vi "Autonomous.vi"   [LabVIEW 2023]
doc: "This VI starts when autonomous period begins, and will automatically be terminated when it ends. You can carry out timed or sensor driven operations directly to I/O or to subsystems without needing to return to the caller."
uses:
  <vilib>/Rock Robotics/WPI/ThirdParty/JAS_Junk/TrajLib/Trajectory_Library.lvlib
  <vilib>/Rock Robotics/WPI/ThirdParty/MJansen/PathPlanner/PathPlanner24.lvlib
  <vilib>/Rock Robotics/WPI/ThirdParty/JAS_Junk/TrajLib/TypeDef/CHASSIS_SPEEDS.ctl
  <vilib>/Rock Robotics/Network Tables/NT Read String.vi
types:
  T1 = typedef "Trajectory_Library.lvlib/CHASSIS_SPEEDS.ctl" = cluster{"vX":dbl, "vY":dbl, "vOmega":dbl}
  T2 = typedef "WPI_JoystickDevRef.ctl" = cluster{"Device":T3}
  T3 = typedef "WPI_JoystickDeviceEnum.ctl" = enum16{"USB 0", "USB 1", "USB 2", "USB 3", "USB 4", "USB 5"}
  T4 = typedef "WPI_MotorControlDeviceRef.ctl" = cluster{"DeviceStatus":errorcluster, "Type":T5, "PWM":cluster{"PWM Channel":T6, "DeadBand":T7}, "CAN":cluster{"Device Number":u8, "SetOutput VI Ref":variant, "GetOutput VI Ref":variant, "Enable VI Ref":variant, "Disable VI Ref":variant, "Data":variant}, "Invert":bool, "DIO PWM":cluster{"PWM \"Enable\" Channel":T6, "DIOChannel":T8, "PWM Rate":dbl}}
  T5 = typedef "WPI_MotorControlType.ctl" = enum16{"PWM", "CAN", "DIO PWM"}
  T6 = typedef "FPGA_DIOPWMChannel.ctl" = enum8{"PWM 0", "PWM 1", "PWM 2", "PWM 3", "PWM 4", "PWM 5", "PWM 6", "PWM 7", "PWM 8", "PWM 9", "PWM MXP 0", "PWM MXP 1", "PWM MXP 2", "PWM MXP 3", "PWM MXP 4", "PWM MXP 5", "PWM MXP 6", "PWM MXP 7", "PWM MXP 8", "PWM MXP 9", "Invalid"}
  T7 = typedef "WPI_PWMDeadband.ctl" = cluster{"Name":string, "maxPositivePwm":i32, "minPositivePwm":i32, "centerPwm":i32, "maxNegativePwm":i32, "minNegativePwm":i32, "angularRange":u16}
  T8 = typedef "FPGA_DIOChannel.ctl" = enum8{"DIO 0", "DIO 1", "DIO 2", "DIO 3", "DIO 4", "DIO 5", "DIO 6", "DIO 7", "DIO 8", "DIO 9", "DIO MXP 0", "DIO MXP 1", "DIO MXP 2", "DIO MXP 3", "DIO MXP 4", "DIO MXP 5", "DIO MXP 6", "DIO MXP 7", "DIO MXP 8", "DIO MXP 9", "DIO MXP 10", "DIO MXP 11", "DIO MXP 12", "DIO MXP 13", "DIO MXP 14", "DIO MXP 15", "SPI Port CS1", "SPI Port CS2", "SPI Port CS3", "SPI Port MISO", "SPI Port MOSI", "Invalid"}
  T9 = typedef "Trajectory_Library.lvlib/ROTATION2D.ctl" = cluster{"VALUE":dbl, "COS":dbl, "SIN":dbl}
  T10 = typedef "Trajectory_Library.lvlib/SWERVE_DRIVE_MODULE_POSITION.ctl" = cluster{"Distance":dbl, "Angle":T9, "P":bool}
  T11 = typedef "PathPlanner24.lvlib/PathPlannerPath.ctl" = cluster{"BezierPoints":T12[], "PreviewStartingRotation":T9, "Reversed":bool, "RotationTargets":T13[], "ConstraintZones":T14[], "EventMarkers":T16[], "GlobalConstraints":T15, "GoalEndState":T19, "AllPoints":T20[]}
  T12 = typedef "Trajectory_Library.lvlib/TRANSLATION2D.ctl" = cluster{"X":dbl, "Y":dbl}
  T13 = typedef "PathPlanner24.lvlib/PathPlannerRotationTarget.ctl" = cluster{"target":T9, "WaypointRelativePosition":dbl, "Exists":bool}
  T14 = typedef "PathPlanner24.lvlib/PathPlannerConstraintsZone.ctl" = cluster{"minWaypointPos":dbl, "maxWaypointPos":dbl, "Constraints":T15, "Present":bool}
  T15 = typedef "PathPlanner24.lvlib/PathPlannerPathConstraints.ctl" = cluster{"MaxVelocityMps;":dbl, "MaxAccelerationMpsSq;":dbl, "MaxAngularVelRadPsEc;":dbl, "MaxAngularAccRadPSecSq":dbl, "Exists":bool}
  T16 = typedef "PathPlanner24.lvlib/PathPlannerEventMarker.ctl" = cluster{"WaypointRelativePos":dbl, "minimumTriggerDistance":dbl, "markerPos":T12, "lastRobotPos":T12, "Command":T17, "markerPos Exists":bool, "LastRobotPoseExists":bool, "Triggered":bool}
  T17 = typedef "PathPlanner24.lvlib/PathPlannerCommandUtil.ctl" = cluster{"waitTime":dbl, "name":string, "pathName":string, "commands":cluster{"type":T18, "waitTime":dbl, "name":string, "pathName":string}[], "type":T18}
  T18 = typedef "PathPlanner24.lvlib/PathPlanner_CommandUtilType_ENUM.ctl" = enum16{"Unknown", "Wait", "Named", "Path", "Sequential", "Parallel", "Race", "Deadline"}
  T19 = typedef "PathPlanner24.lvlib/PathPlannerGoalEndState.ctl" = cluster{"Velocity":dbl, "Rotation":T9}
  T20 = typedef "PathPlanner24.lvlib/PathPlannerPathPoint.ctl" = cluster{"Position":T12, "HolonomicRotation":T9, "DistAlongPath":dbl, "CurveRadius":dbl, "MaxV":dbl, "Constraints":T15, "HolonomicRotationExists":bool}
  T21 = typedef "ADIS16470 Device Reference.ctl" = cluster{"DevStatus":errorcluster, "Hardware Config":T22, "Calibration Complete":refnum<notifier>, "Status Reference":refnum<data-value>, "Data Reference":refnum<data-value>, "Sychronous Process VI":T25, "Cmd FIFO":refnum<k33>, "Source":T26, "Data FIFO":refnum<k33>, "Calibration Time (ms)":u32, "Data Reference":refnum<data-value>}
  T22 = typedef "ADIS16470 Hardware Configuration.ctl" = cluster{"SPI Clock Rate (Hz)":dbl, "IMU SPI Mode (3)":T23, "IMU Reset Pin":T8, "IMU SPI Bus":T24, "IMU Data Ready Pin":T8, "Stall Config":cluster{"Pow2BytesPerRead":u8, "StallTicks":u16, "CsToSclkTicks":u8}}
  T23 = typedef "WPI_SPIMode.ctl" = enum16{"Mode 0 (Clk Idle Low,Sample on Leading)", "Mode 1 (Clk Idle Low,Sample on Trailing)", "Mode 2 (Clk Idle High,Sample on Leading)", "Mode 3 (Clk Idle High,Sample on Trailing)"}
  T24 = typedef "spi_bus.ctl" = enum16{"SPI On-Board, CS0", "SPI On-Board, CS1", "SPI On-Board, CS2", "SPI On-Board, CS3", "SPI MXP", "Invalid"}
  T25 = typedef "ADIS16470 Process.ctl" = refnum<vi>
  T26 = typedef "FPGA_CounterEncoderSourceConvertionLVSourceType.ctl" = cluster{"DevStatus":errorcluster, "AnalogTriggerMode?":bool, "DigitalMode":cluster{"DIO Channel":T27}, "AnalogTriggerMode":cluster{"AnalogTriggerIndex":T28, "OutputType":T29}}
  T27 = typedef "FPGA_DIODigitalSourceChannel.ctl" = enum8{"DIO 0", "DIO 1", "DIO 2", "DIO 3", "DIO 4", "DIO 5", "DIO 6", "DIO 7", "DIO 8", "DIO 9", "DIO MXP 0", "DIO MXP 1", "DIO MXP 2", "DIO MXP 3", "DIO MXP 4", "DIO MXP 5", "DIO MXP 6", "DIO MXP 7", "DIO MXP 8", "DIO MXP 9", "DIO MXP 10", "DIO MXP 11", "DIO MXP 12", "DIO MXP 13", "DIO MXP 14", "DIO MXP 15", "SPI Port CS1", "SPI Port CS2", "SPI Port CS3", "SPI Port MISO", "SPI Port MOSI", "Disabled"}
  T28 = typedef "FPGA_AnalogTriggerIndex.ctl" = enum8{"Trig 0", "Trig 1", "Trig 2", "Trig 3", "Trig 4", "Trig 5", "Trig 6", "Trig 7", "Invalid"}
  T29 = typedef "FPGA_AnalogTriggerOutType.ctl" = enum16{"InWindow", "TriggerState", "Rising", "Falling"}
  T30 = typedef "ADIS16470 Data.ctl" = cluster{"XAngle":dbl, "YAngle":dbl, "ZAngle":dbl}
  T31 = typedef "Trajectory_Library.lvlib/POSE2D.ctl" = cluster{"TRANSLATION":T12, "ROTATION":T9}
  T32 = typedef "Trajectory_Library.lvlib/SWERVE_DRIVE_KINEMATICS.ctl" = cluster{"NumModules":i32, "InverseKinematics":T33, "ForwardKinematics":T33, "Modules":T12[], "PrevCoR":T12, "SavedModuleStates":T34[]}
  T33 = typedef "NI_Matrix.lvlib/RealMatrix.ctl" = dbl[][]
  T34 = typedef "Trajectory_Library.lvlib/SWERVE_DRIVE_MODULE_STATE.ctl" = cluster{"Speed":dbl, "Angle":T9}
  T35 = typedef "Trajectory_Library.lvlib/SWERVE_DRIVE_ODOMETRY.ctl" = cluster{"POSE":T31, "GyroOffset":T9, "PreviousAngle":T9, "PrevModulePositions":T10[], "NumModules":i32}
  T36 = typedef "Trajectory_Library.lvlib/PID_TUNING.ctl" = cluster{"Kp":dbl, "Ki":dbl, "Kd":dbl, "MaximumIntegral":dbl, "MinimumIntegral":dbl, "IntegralZone":dbl}
  T37 = typedef "Trajectory_Library.lvlib/PROFILED_PID_CONTROLLER.ctl" = cluster{"Controller":T38, "Goal":T39, "Setpoint":T39, "Constraint":T40}
  T38 = typedef "Trajectory_Library.lvlib/PID_CONTROLLER.ctl" = cluster{"Kp":dbl, "Ki":dbl, "Kd":dbl, "Period":dbl, "Max_Integral":dbl, "Min_Integral":dbl, "Max_Input":dbl, "Min_Input":dbl, "Continuous":bool, "PositionError":dbl, "VelocityError":dbl, "PrevError":dbl, "Total_Integral":dbl, "PositionTolerance":dbl, "VelocityTolerance":dbl, "SetPoint":dbl, "Kf":dbl, "Prev_Deriv":dbl, "Prev_Deriv 2":dbl, "DerivativeFilter":bool, "Min_Output":dbl, "Max_Output":dbl, "Prev_F_P":dbl, "Prev_F_P_2":dbl, "AntiWindupActive":bool, "Measurement":dbl, "IntegralZone":dbl}
  T39 = typedef "Trajectory_Library.lvlib/TRAPEZOID_PROFILE_STATE.ctl" = cluster{"Position":dbl, "Velocity":dbl}
  T40 = typedef "Trajectory_Library.lvlib/TRAPEZOID_PROFILE_CONSTRAINT.ctl" = cluster{"MaxVelocity":dbl, "MaxAcceleration":dbl}
  T41 = typedef "PathPlanner24.lvlib/PathPlannerReplanningConfig.ctl" = cluster{"enableInitialReplanning":bool, "enableDynamicReplanning":bool, "dynamicReplanningTotalErrorThreshold":dbl, "dynamicReplanningErrorSpikeThreshold":dbl}
  T42 = typedef "Trajectory_Library.lvlib/HOLONOMIC_PACK_TUNING.ctl" = cluster{"X PID Tuning":T36, "Y PID Tuning":T36, "thetaProfiledPID_CTRL":T37}
  T43 = typedef "PathPlanner24.lvlib/PathPlannerCmdFollowHolConfig.ctl" = cluster{"HOLONOMIC_CTRL_PACK_TUNING":T42, "Max Wheel Speed M/S":dbl, "Tolerance SI":T31, "Drive Base Radius M":dbl, "ControlPastEnd_Sec":dbl, "ReplanningConfig":T41, "Period_Sec":dbl, "Trigger Events":bool}
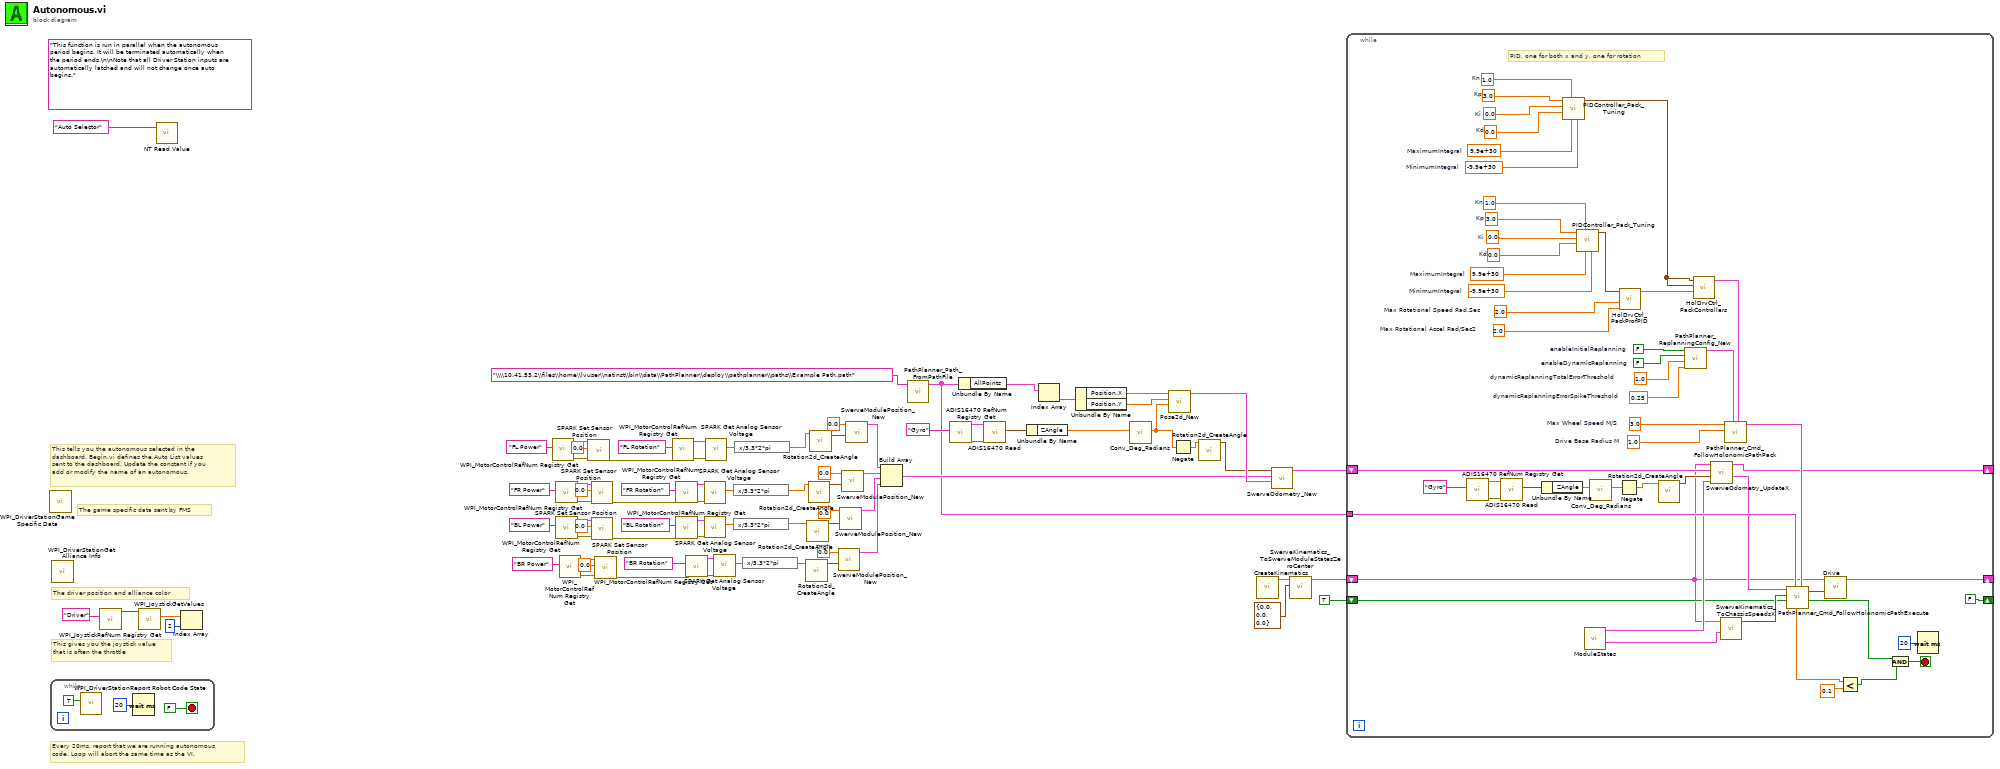
[diagram p0: block diagram]
diagram:
  (unwired) "This function is run in parallel when the autonomous period begins. It will be terminated automatically when the period ends.\n\nNote that all Driver Station inputs are automatically latched and will not change once auto begins."
  # "The game specific data sent by FMS"
  # "This tells you the autonomous selected in the \ndashboard. Begin.vi defines the Auto List values\nsent to the dashboard. Update the constant if you\nadd or modify the name of an autonomous."
  # "Every 20ms, report that we are running autonomous\ncode. Loop will abort the same time as the VI."
  # "This gives you the joystick value\nthat is often the throttle"
  # "The driver position and alliance color"
  n1 = call <vilib>:"WPI_DriverStationGame Specific Data.vi"() -> ()  [unwired: 11 in, 1 out]
  n2 = while {
    stop <- FALSE stop-if-true
    n3 = call <vilib>:"WPI_DriverStationReport Robot Code State.vi"("Autonomous"=TRUE) -> ()  [unwired: 10 in, 1 out]
    n4 = Wait (ms)(milliseconds to wait=u32 20) -> ()  [unwired: 1 out]
  }
  n5 = call <vilib>:"WPI_DriverStationGet Alliance Info.vi"() -> ()  [unwired: 12 out]
  n6 = call <vilib>:"WPI_JoystickRefNum Registry Get.vi"("refnum name"="Driver") -> ("JoystickDevRef"=w77:T2)  [unwired: 1 in, 9 out]
  n7 = call <vilib>:"WPI_JoystickGetValues.vi"("JoystickDevRef"=w77) -> ("Axes"=w76:dbl[])  [unwired: 6 in, 4 out]
  n8 = call-poly <vilib>:"NT Read Value.vi"("name"="Auto Selector" ("Name")) -> ()  [unwired: 8 in, 3 out]
  n9 = Index Array(array=w76, index=2) -> ()  [unwired: 1 out]
  n10 = call <vilib>:"WPI_MotorControlRefNum Registry Get.vi"("refnum name"="FL Power") -> ("error out"=w72:errorcluster, "MotorControlDevRef"=w71:T4)  [unwired: 9 in]
  n11 = call <vilib>:"WPI_MotorControlRefNum Registry Get.vi"("refnum name"="FR Power") -> ("error out"=w67:errorcluster, "MotorControlDevRef"=w68:T4)  [unwired: 9 in]
  n12 = call <vilib>:"WPI_MotorControlRefNum Registry Get.vi"("refnum name"="BL Power") -> ("error out"=w64:errorcluster, "MotorControlDevRef"=w63:T4)  [unwired: 9 in]
  n13 = call <vilib>:"WPI_MotorControlRefNum Registry Get.vi"("refnum name"="BR Power") -> ("error out"=w59:errorcluster, "MotorControlDevRef"=w60:T4)  [unwired: 9 in]
  n14 = call <vilib>:"SPARK Set Sensor Position.vi"("error in"=w72, "Position"=0.0, "MotorControlDeviceRef"=w71) -> ("error out"=w53:errorcluster)  [unwired: 7 in, 1 out]
  n15 = call <vilib>:"SPARK Set Sensor Position.vi"("error in"=w67, "Position"=0.0, "MotorControlDeviceRef"=w68) -> ("error out"=w52:errorcluster)  [unwired: 7 in, 1 out]
  n16 = call <vilib>:"SPARK Set Sensor Position.vi"("error in"=w64, "Position"=0.0, "MotorControlDeviceRef"=w63) -> ("error out"=w51:errorcluster)  [unwired: 7 in, 1 out]
  n17 = call <vilib>:"SPARK Set Sensor Position.vi"("error in"=w59, "Position"=0.0, "MotorControlDeviceRef"=w60) -> ("error out"=w50:errorcluster)  [unwired: 7 in, 1 out]
  n18 = call <vilib>:"WPI_MotorControlRefNum Registry Get.vi"("error in (no error)"=w53, "refnum name"="FL Rotation") -> ("error out"=w49:errorcluster, "MotorControlDevRef"=w48:T4)  [unwired: 8 in]
  n19 = call <vilib>:"WPI_MotorControlRefNum Registry Get.vi"("error in (no error)"=w52, "refnum name"="FR Rotation") -> ("error out"=w47:errorcluster, "MotorControlDevRef"=w46:T4)  [unwired: 8 in]
  n20 = call <vilib>:"WPI_MotorControlRefNum Registry Get.vi"("error in (no error)"=w51, "refnum name"="BL Rotation") -> ("error out"=w45:errorcluster, "MotorControlDevRef"=w44:T4)  [unwired: 8 in]
  n21 = call <vilib>:"WPI_MotorControlRefNum Registry Get.vi"("error in (no error)"=w50, "refnum name"="BR Rotation") -> ("error out"=w43:errorcluster, "MotorControlDevRef"=w42:T4)  [unwired: 8 in]
  n22 = call <vilib>:"SPARK Get Analog Sensor Voltage.vi"("error in (no error)"=w47, "MotorControlDevRef in"=w46) -> ("Analog Sensor Voltage"=w39:dbl)  [unwired: 6 in, 3 out]
  n23 = call <vilib>:"SPARK Get Analog Sensor Voltage.vi"("error in (no error)"=w45, "MotorControlDevRef in"=w44) -> ("Analog Sensor Voltage"=w40:dbl)  [unwired: 6 in, 3 out]
  n24 = call <vilib>:"SPARK Get Analog Sensor Voltage.vi"("error in (no error)"=w49, "MotorControlDevRef in"=w48) -> ("Analog Sensor Voltage"=w38:dbl)  [unwired: 6 in, 3 out]
  n25 = call <vilib>:"SPARK Get Analog Sensor Voltage.vi"("error in (no error)"=w43, "MotorControlDevRef in"=w42) -> ("Analog Sensor Voltage"=w41:dbl)  [unwired: 6 in, 3 out]
  n26 = expression code="x/3.3*2*pi"(w39) -> (w36:dbl)
  n27 = expression code="x/3.3*2*pi"(w40) -> (w35:dbl)
  n28 = expression code="x/3.3*2*pi"(w38) -> (w37:dbl)
  n29 = expression code="x/3.3*2*pi"(w41) -> (w34:dbl)
  n30 = call <vilib>:"Rotation2d_CreateAngle.vi"("Angle"=w34) -> ("ROTATION"=w28:T9)  [unwired: 10 in]
  n31 = call <vilib>:"Rotation2d_CreateAngle.vi"("Angle"=w35) -> ("ROTATION"=w29:T9)  [unwired: 10 in]
  n32 = call <vilib>:"Rotation2d_CreateAngle.vi"("Angle"=w36) -> ("ROTATION"=w30:T9)  [unwired: 10 in]
  n33 = call <vilib>:"Rotation2d_CreateAngle.vi"("Angle"=w37) -> ("ROTATION"=w33:T9)  [unwired: 10 in]
  n34 = call <vilib>:"SwerveModulePosition_New.vi"("ROTATION"=w28, "Distance"=0.0) -> ("SWERVE_DRIVE_MODULE_POSITION"=w22:T10)  [unwired: 9 in]
  n35 = call <vilib>:"SwerveModulePosition_New.vi"("ROTATION"=w29, "Distance"=0.0) -> ("SWERVE_DRIVE_MODULE_POSITION"=w23:T10)  [unwired: 9 in]
  n36 = call <vilib>:"SwerveModulePosition_New.vi"("ROTATION"=w30, "Distance"=0.0) -> ("SWERVE_DRIVE_MODULE_POSITION"=w24:T10)  [unwired: 9 in]
  n37 = call <vilib>:"SwerveModulePosition_New.vi"("ROTATION"=w33, "Distance"=0.0) -> ("SWERVE_DRIVE_MODULE_POSITION"=w25:T10)  [unwired: 9 in]
  n38 = Build Array(w25, w24, w23, w22) -> (w7:T10[])
  n39 = call <vilib>:"PathPlanner_Path_FromPathFile.vi"("FileName"="\\\\10.41.53.2\\files\\home\\lvuser\\natinst\\bin\\data\\PathPlanner\\deploy\\pathplanner\\paths\\Example Path.path" ("Path")) -> ("PathPlannerPath"=w2:T11)  [unwired: 8 in, 2 out]
  n40 = call <vilib>:"ADIS16470 RefNum Registry Get.vi"("refnum name"="Gyro") -> ("error out"=w20:errorcluster, "ADIS16470DevRef out"=w19:T21)  [unwired: 9 in]
  n41 = Unbundle By Name(w2) -> ("AllPoints"=w15:T20[])
  n42 = call <vilib>:"ADIS16470 Read.vi"("error in (no error)"=w20, "ADIS16470DevRef"=w19) -> ("ADIS16470 Value"=w17:T30)  [unwired: 6 in, 3 out]
  n43 = Unbundle By Name(w17) -> ("ZAngle"=w16:dbl)
  n44 = Index Array(array=w15) -> (element=w14:T20)  [unwired: 1 in]
  n45 = Unbundle By Name(w14) -> ("Position.X"=w12:dbl, "Position.Y"=w13:dbl)
  n46 = call <vilib>:"Conv_Deg_Radians.vi"("Degress"=w16) -> ("Radians"=w11:dbl)  [unwired: 10 in]
  n47 = call <vilib>:"Pose2d_New.vi"("Heading"=w11, "Y"=w13, "X"=w12) -> ("out POSe"=w9:T31)  [unwired: 8 in]
  n48 = Negate(x=w11) -> (-x=w10:dbl)
  n49 = call <vilib>:"Rotation2d_CreateAngle.vi"("Angle"=w10) -> ("ROTATION"=w8:T9)  [unwired: 10 in]
  n50 = call "CreateKinematics.vi"() -> ("SWERVE_DRIVE_KINEMATICS"=w1:T32)  [unwired: 11 in]
  n51 = call <vilib>:"SwerveOdometry_New.vi"("InitialPose"=w9, "Module Positions"=w7, "gyroAngle"=w8) -> ("SWERVE_DRIVE_ODOMETRY"=w4:T35)  [unwired: 8 in]
  n52 = call <vilib>:"SwerveKinematics_ToSwerveModuleStatesZeroCenter.vi"("ChassisSpeeds"=T1 {"vX"=0.0, "vY"=0.0, "vOmega"=0.0} ("CHASSIS"), "in SWERVE_DRIVE_KINEMATICS"=w1) -> ("out SWERVE_DRIVE_KINEMATICS"=w3:T32)  [unwired: 8 in, 1 out]
  n53 = while {
    shift-right: [FALSE ("Reset")] -> _
    shift-left: TRUE ("Reset") -> [w86]
    shift-right: [w84] -> _
    shift-left: w4 -> [w126]
    tunnel: w2 -> [w117]
    shift-right: [w83] -> _
    shift-left: w3 -> [w82]
    stop <- w128 stop-if-true
    w112 = FALSE  # enableInitialReplanning
    w111 = FALSE  # enableDynamicReplanning
    w110 = 1.0  # dynamicReplanningTotalErrorThreshold
    w109 = 0.25  # dynamicReplanningErrorSpikeThreshold
    w114 = 1.0  # Drive Base Radius M
    w113 = 3.0  # Max Wheel Speed M/S
    w101 = 1.0  # Kn
    w99 = 3.0  # Kp
    w94 = 0.0  # Ki
    w93 = 0.0  # Kd
    w92 = 9.9e+30  # MaximumIntegral
    w91 = -9.9e+30  # MinimumIntegral
    w102 = 1.0  # Kn
    w100 = 3.0  # Kp
    w98 = 0.0  # Ki
    w97 = 0.0  # Kd
    w96 = 9.9e+30  # MaximumIntegral
    w95 = -9.9e+30  # MinimumIntegral
    w103 = 2.0  # Max Rotational Accel Rad/Sec2
    w104 = 2.0  # Max Rotational Speed Rad.Sec
    # "PID, one for both x and y, one for rotation"
    n54 = call <vilib>:"ADIS16470 RefNum Registry Get.vi"("refnum name"="Gyro") -> ("error out"=w122:errorcluster, "ADIS16470DevRef out"=w123:T21)  [unwired: 9 in]
    n55 = call <vilib>:"ADIS16470 Read.vi"("error in (no error)"=w122, "ADIS16470DevRef"=w123) -> ("ADIS16470 Value"=w125:T30)  [unwired: 6 in, 3 out]
    n56 = Unbundle By Name(w125) -> ("ZAngle"=w121:dbl)
    n57 = call <vilib>:"PIDController_Pack_Tuning.vi"("MinimumIntegral"=w95, "MaximumIntegral"=w96, "Kn"=w102, "Kd"=w97, "Ki"=w98, "Kp"=w100) -> ("PID Tuning"=w90:T36)  [unwired: 5 in]
    n58 = call <vilib>:"PIDController_Pack_Tuning.vi"("MinimumIntegral"=w91, "MaximumIntegral"=w92, "Kn"=w101, "Kd"=w93, "Ki"=w94, "Kp"=w99) -> ("PID Tuning"=w105:T36)  [unwired: 5 in]
    n59 = call "ModuleStates.vi"() -> ("Module States"=w87:cluster{"Meters":dbl, "ROTATION":T9}[], "Module Positions"=w88:T10[])  [unwired: 10 in]
    n60 = call <vilib>:"Conv_Deg_Radians.vi"("Degress"=w121) -> ("Radians"=w120:dbl)  [unwired: 10 in]
    n61 = Negate(x=w120) -> (-x=w119:dbl)
    n62 = call <vilib>:"HolDrvCtrl_PackProfPID.vi"("Max Accel"=w103, "Max Speed"=w104, "Theta PID Tuning"=w105) -> ("Theta PID CONTROLLER"=w107:T37)  [unwired: 8 in]
    n63 = call <vilib>:"Rotation2d_CreateAngle.vi"("Angle"=w119) -> ("ROTATION"=w118:T9)  [unwired: 10 in]
    n64 = call <vilib>:"PathPlanner_ReplanningConfig_New.vi"("dynamicReplanningErrorSpikeThreshold"=w109, "dynamicReplanningTotalErrorThreshold"=w110, "enableDynamicReplanning"=w111, "enableInitialReplanning"=w112) -> ("ReplanningConfig"=w108:T41)  [unwired: 7 in]
    n65 = call <vilib>:"HolDrvCtrl_PackControllers.vi"("thetaProfiledPID_CTRL"=w107, "Y PID Tuning"=w90, "X PID Tuning"=w90) -> ("HOLONOMIC_CTRL_PACK_TUNING"=w106:T42)  [unwired: 8 in]
    n66 = call <vilib>:"SwerveOdometry_UpdateX.vi"("module Positions"=w88, "gyroAngle"=w118, "in SWERVE_DRIVE_ODOMETRY"=w126, "SWERVE_DRIVE_KINEMATICS"=w82) -> ("robot POSE"=w116:T31, "out SWERVE_DRIVE_ODOMETRY"=w84:T35)  [unwired: 5 in, 1 out]
    n67 = call <vilib>:"SwerveKinematics_ToChassisSpeedsX.vi"("WheelStates"=w87, "in SWERVE_DRIVE_KINEMATICS"=w82) -> ("Chassis Speed"=w115:T1)  [unwired: 9 in]
    n68 = call <vilib>:"PathPlanner_Cmd_FollowHolonomicPathPack.vi"("HOLONOMIC_CTRL_PACK_TUNING"=w106, "ReplanningConfig"=w108, "Drive Base Radius M"=w114, "Max Wheel Speed M/S"=w113) -> ("PathPlanner_Ctrl_HolDrvConfig"=w89:T43)  [unwired: 7 in]
    n69 = call <vilib>:"PathPlanner_Cmd_FollowHolonomicPathExecute.vi"("PathPlanner_Cmd_FollowHolConfig"=w89, "PathPlannerPath"=w117, "Reset"=w86, "CurrentChassisSpeeds"=w115, "Current Pose SI"=w116) -> ("Position Error M"=w127:dbl, "Complete"=w129:bool, "calcChassisSpeed"=w133:T1)  [unwired: 2 in, 2 out]
    n70 = call "Drive.vi"("CHASSIS"=w133, "SWERVE_DRIVE_KINEMATICS"=w82) -> ("out SWERVE_DRIVE_KINEMATICS"=w83:T32)  [unwired: 8 in, 1 out]
    n71 = Less?(x=w127, y=0.1) -> (x < y?=w130:bool)
    n72 = And(x=w129, y=w130) -> (x .and. y?=w128:bool)
    n73 = Wait (ms)(milliseconds to wait=u32 20) -> ()  [unwired: 1 out]
  }
